vi "Write Value.vi"(8 "error in (no error)":errorcluster, 10 "Value":sgl, 11 "float in":refnum<class "float.lvclass">) -> (0 "error out":errorcluster, 3 "float out":refnum<class "float.lvclass">)   [LabVIEW 2020, in "Protobuf RAW.lvlib" / "float.lvclass"]
uses:
  float.lvclass
  float.lvclass/float.ctl
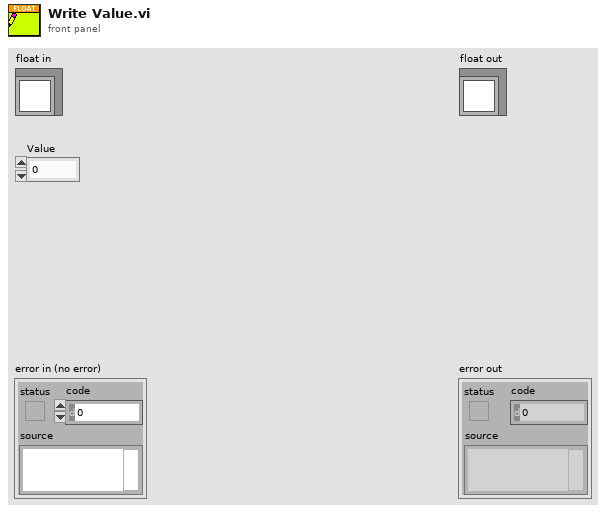
[diagram p1: front panel]
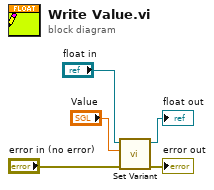
[diagram p0: block diagram]
diagram:
  n1 = call-dynamic "Set Variant.vi"("error in (no error)"="error in (no error)", "Value"="Value", "Proto Type Common in"="float in") -> ("error out"=→"error out":errorcluster, "Proto Type Common out"=→"float out":refnum<class "float.lvclass">)  [unwired: 7 in]
